vi "generate video name.vi"(11 "video info":T1 {"date" format="%<%x>T"}) -> (3 "date+model":string)   [LabVIEW 2023, in "File Classes.lvlib" / "Video File.lvclass"]
uses:
  Video File.lvclass
  Controls/video exif info cluster.ctl
  File Classes.lvlib
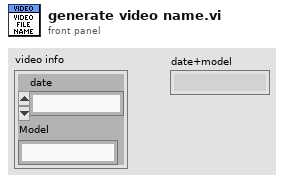
[diagram p1: front panel]
types:
  T1 = typedef "File Classes.lvlib/video exif info cluster.ctl" = cluster{"date":timestamp, "Model":string}
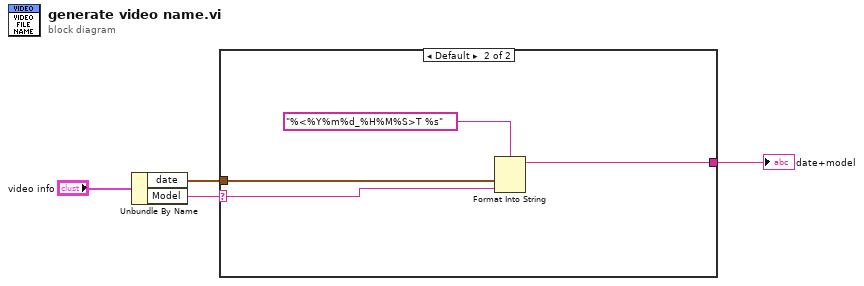
[diagram p0: block diagram]
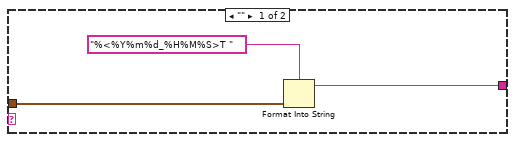
[diagram p2: hidden frame]
diagram:
  n1 = Unbundle By Name("video info") -> ("date"=w2:timestamp, "Model"=w3:string)
  n2 = case shown="Default" w3 {
    selector: w3 -> [_ w8]
    tunnel: w2 -> [w7 w11]
    tunnel: [w5 w9] -> w1
    frame "" {
      n3 = Format Into String(format string="%<%Y%m%d_%H%M%S>T " ("time format string (%c)"), w7) -> (resulting string=w5:string)  [unwired: 2 in, 1 out]
    }
    frame Default {
      n4 = Format Into String(format string="%<%Y%m%d_%H%M%S>T %s" ("time format string (%c)"), w11, w8) -> (resulting string=w9:string)  [unwired: 2 in, 1 out]
    }
  }
  "date+model" <- w1
